vi "Read (Multiple Points).vi"(0 "VISA resource name":refnum<visa-resource-name>, 1 "Sample Count (1)":i32=1, 5 "Timeout (10000 ms)":i32=10000 format="%#.6g", 11 "error in (no error)":errorcluster, 12 "Output Mode (0: Fixed)":u16(ring) items=["Fixed", "Sweep", "List"]) -> (3 "Voltage":sgl[](array[numeric]), 4 "VISA resource name out":refnum<visa-resource-name>, 6 "Current":sgl[](array[numeric]), 8 "Resistance":sgl[](array[numeric]), 10 "Timestamp":sgl[](array[numeric]), 14 "Status":sgl[](array[numeric]), 15 "error out":errorcluster)   [LabVIEW 2012, in "Keithley 24XX.lvlib"]
doc: "Initiates an acquisition and returnes the raw data gathered from the instrument."
uses:
  <instrlib>/Keithley 24XX/Keithley 24XX.lvlib
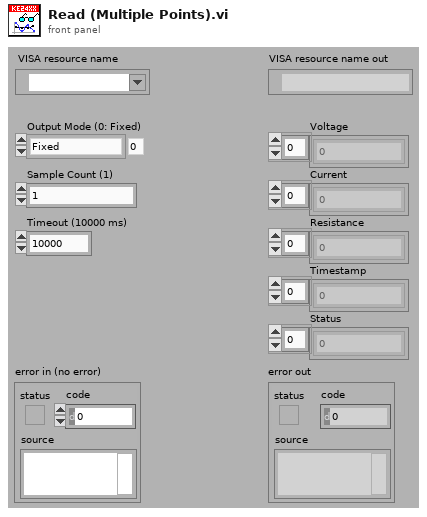
[diagram p1: front panel]
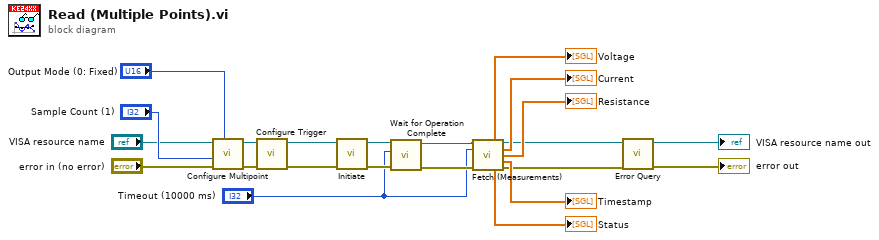
[diagram p0: block diagram]
diagram:
  n1 = call <instrlib>:"Configure Multipoint.vi"("Output Mode (0: Fixed)"="Output Mode (0: Fixed)", "error in (no error)"="error in (no error)", "Trigger Count (1)"="Sample Count (1)", "VISA resource name"="VISA resource name") -> ("error out"=w9:errorcluster, "VISA resource name out"=w10:refnum<visa-resource-name>)  [unwired: 6 in]
  n2 = call <instrlib>:"Configure Trigger.vi"("error in (no error)"=w9, "VISA resource name"=w10) -> ("error out"=w1:errorcluster, "VISA resource name out"=w2:refnum<visa-resource-name>)  [unwired: 8 in]
  n3 = call <instrlib>:"Initiate.vi"("error in (no error)"=w1, "VISA resource name"=w2) -> ("error out"=w14:errorcluster, "VISA resource name out"=w15:refnum<visa-resource-name>)  [unwired: 8 in]
  n4 = call <instrlib>:"Wait for Operation Complete.vi"("error in (no error)"=w14, "Timeout (10000 ms)"="Timeout (10000 ms)", "VISA resource name"=w15) -> ("error out"=w13:errorcluster, "VISA resource name out"=w12:refnum<visa-resource-name>)  [unwired: 7 in]
  n5 = call <instrlib>:"Fetch (Measurements).vi"("VISA resource name"=w12, "Timeout (10000 ms)"="Timeout (10000 ms)", "error in (no error)"=w13) -> ("Voltage"=→"Voltage":sgl[], "VISA resource name out"=w4:refnum<visa-resource-name>, "Current"=→"Current":sgl[], "Resistance"=→"Resistance":sgl[], "Timestamp"=→"Timestamp":sgl[], "Status"=→"Status":sgl[], "error out"=w3:errorcluster)  [unwired: 6 in]
  n6 = call <instrlib>:"Error Query.vi"("error in (no error)"=w3, "VISA resource name"=w4) -> ("error out"=→"error out":errorcluster, "VISA resource name out"=→"VISA resource name out":refnum<visa-resource-name>)  [unwired: 6 in, 2 out]
